vi "Read display name.vi"(8 "error in":errorcluster, 11 "module editor node in":refnum<class "module editor node.lvclass">) -> (0 "error out":errorcluster, 2 "display name":string, 3 "module editor node out":refnum<class "module editor node.lvclass">)   [LabVIEW 2013, in "PL Framework Configuration Tool.lvlib" / "module editor node.lvclass"]
uses:
  module editor node.lvclass
  <vilib>/NI/Configuration Framework/serializable configuration/NISE_CEF_serializable configuration.lvclass
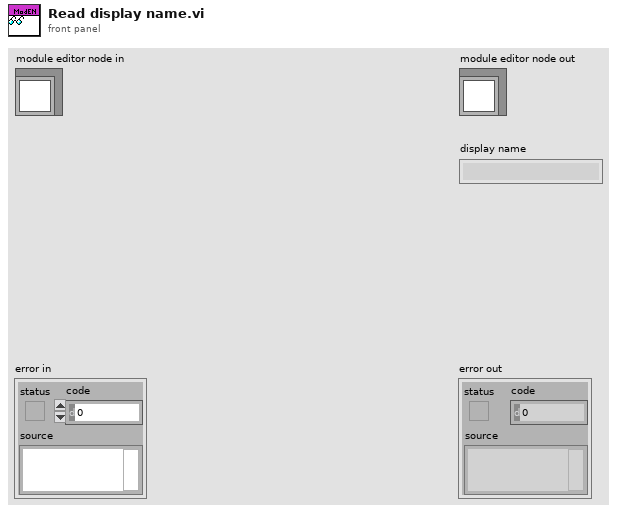
[diagram p1: front panel]
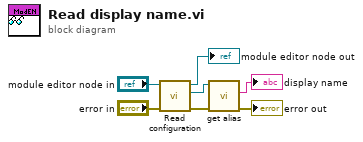
[diagram p0: block diagram]
diagram:
  n1 = call-dynamic "Read configuration.vi"("error in"="error in", "NISE_CEF_serializable node in"="module editor node in") -> ("error out"=w4:errorcluster, "configuration"=w1:refnum<class "NISE_CEF_serializable configuration.lvclass">, "NISE_CEF_serializable node out"=→"module editor node out":refnum<class "module editor node.lvclass">)  [unwired: 7 in]
  n2 = call <vilib>:"get alias.vi"("error in"=w4, "configuration in"=w1) -> ("error out"=→"error out":errorcluster, "alias"=→"display name":string)  [unwired: 7 in, 1 out]
